vi "_CSMObj-Clone Worker.vi"(8 "Error in":errorcluster caption="Error in (no error)", 11 "CSMObj in":T1={"Requested Name"="", "Module Name"="", "Mode"=enum."Stand Alone", "Queue"=refnum, "CSM-Data"=refnum, "User Event"=refnum, "Status Change Event"=refnum, "Allowed Messages"=[], "Mode-Data"=refnum, "Group Name"="", "Exit Event"=refnum}) -> (0 "Error out":errorcluster, 2 "output cluster":T1={"Requested Name"="", "Module Name"="", "Mode"=enum."Stand Alone", "Queue"=refnum, "CSM-Data"=refnum, "User Event"=refnum, "Status Change Event"=refnum, "Allowed Messages"=[], "Mode-Data"=refnum, "Group Name"="", "Exit Event"=refnum}, 3 "CSMObj out":T1={"Requested Name"="", "Module Name"="", "Mode"=enum."Stand Alone", "Queue"=refnum, "CSM-Data"=refnum, "User Event"=refnum, "Status Change Event"=refnum, "Allowed Messages"=[], "Mode-Data"=refnum, "Group Name"="", "Exit Event"=refnum})   [LabVIEW 2020, in "Communicable State Machine.lvlib"]
uses:
  Communicable State Machine.lvlib
  _CSMObj.ctl
  Priority Queue.lvclass
  _CSM_MODE.ctl
  _CSMObj-Data.ctl
  _CSM Status Change Event Data.ctl
  _CSMObj-ModeData.ctl
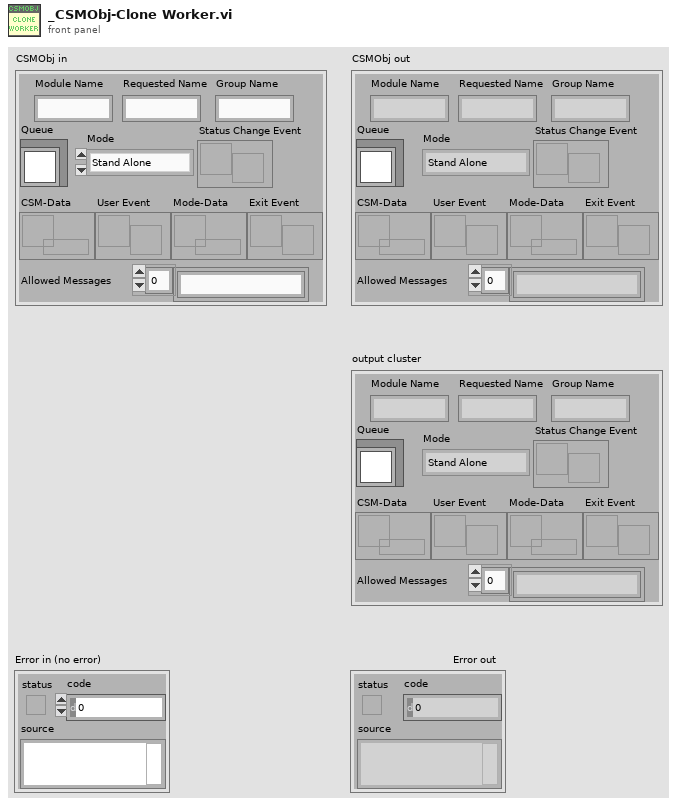
[diagram p1: front panel]
types:
  T1 = typedef "Communicable State Machine.lvlib/_CSMObj.ctl" = cluster{"Requested Name":string, "Module Name":string, "Mode":T2, "Queue":refnum<class "Priority Queue.lvclass">, "CSM-Data":refnum<data-value>, "User Event":refnum<user-event>, "Status Change Event":refnum<user-event>, "Allowed Messages":string[], "Mode-Data":refnum<data-value>, "Group Name":string, "Exit Event":refnum<user-event>}
  T2 = typedef "Communicable State Machine.lvlib/_CSM_MODE.ctl" = enum16{"Not Exist", "Stand Alone", "CSM", "Worker Agent", "Worker", "Chain", "Chain Node"}
  T3 = typedef "Communicable State Machine.lvlib/_CSMObj-Data.ctl" = cluster{"RemoteMessge?":bool, "error":errorcluster}
  T4 = typedef "Communicable State Machine.lvlib/_CSMObj-ModeData.ctl" = cluster{"Share Count":i32, "Messages of Chain Nodes":cluster{"Module Name":string, "Allowed Messages":string[]}[], "Chain Message Mapping Map":variant}
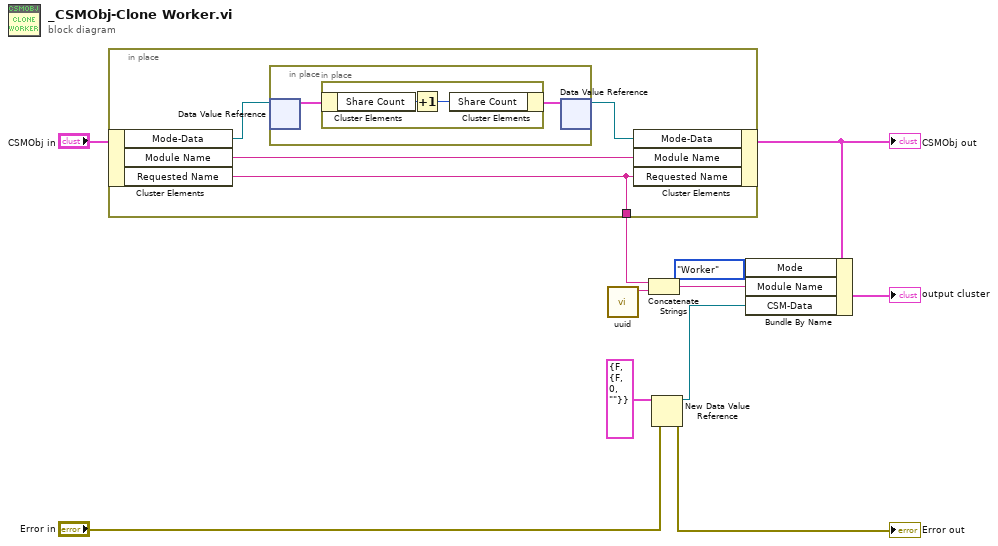
[diagram p0: block diagram]
diagram:
  n1 = in-place "In Place Element Structure" {
    in-place-border: [w14] -> w7
    n2 = in-place-cluster #1("CSMObj in") -> ("Mode-Data"=w12:refnum<data-value>, "Module Name"=w15:string, "Requested Name"=w14:string)
    n3 = in-place {
      n4 = in-place-dvr #2(w12) -> (w17:T4)  [unwired: 1 out]
      n5 = in-place {
        n6 = in-place-cluster #3(w17) -> ("Share Count"=w19:i32)
        n7 = Increment(x=w19) -> (x+1=w18:i32)
        n8 = in-place-cluster #3("Share Count"=w18) -> (w16:T4)
      }
      n9 = in-place-dvr #2(w16) -> (w13:refnum<data-value>)  [unwired: 1 out]
    }
    n10 = in-place-cluster #1("Mode-Data"=w13, "Module Name"=w15, "Requested Name"=w14) -> (w10:T1)
  }
  "CSMObj out" <- w10
  n11 = call "uuid.vi"() -> ("UUID"=w9:string)  [unwired: 11 in]
  n12 = Concatenate Strings(w7, w9) -> (w8:string)
  n13 = New Data Value Reference(data value=T3 {"RemoteMessge?"=FALSE, "error"={"status"=FALSE, "code"=0, "source"=""}} ("CSMObj-Data"), error in="Error in") -> (data value reference=w3:refnum<data-value>, error out=→"Error out":errorcluster)
  n14 = Bundle By Name(cluster=w10, "Mode"=_CSM_MODE."Worker", "Module Name"=w8, "CSM-Data"=w3) -> (→"output cluster":T1)
